vi "Offset by dx and dy.vi"(8 "error in (no error)":errorcluster caption="错误输入（无错误）", 9 "dy":dbl, 10 "dx":dbl, 11 "Point 输入":refnum<class "Point.lvclass"> caption="DNL_LabVIEW Object in") -> (0 "error out":errorcluster caption="错误输出", 3 "Point 输出":refnum<class "Point.lvclass"> caption="DNL_LabVIEW Object out")   [LabVIEW 2011, in "Point.lvclass"]
uses:
  Point.lvclass
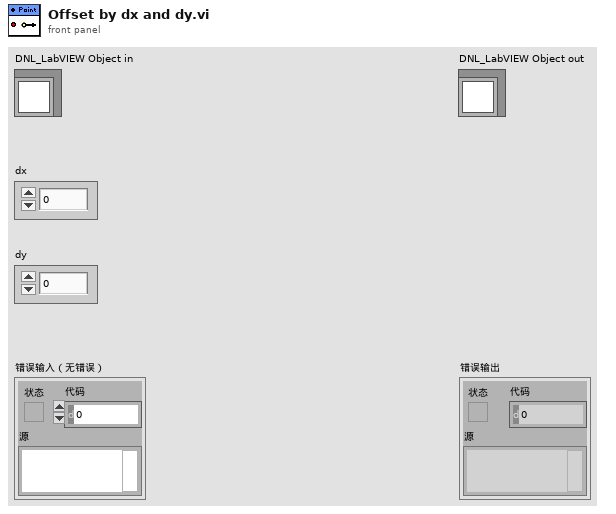
[diagram p1: front panel]
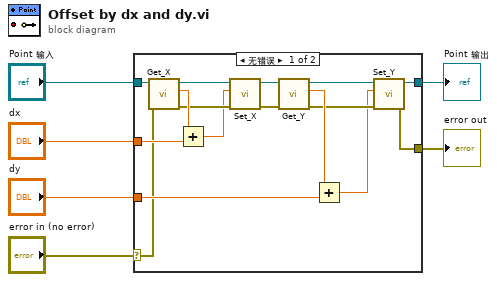
[diagram p0: block diagram]
diagram:
  n1 = case shown="无错误" "error in (no error)" {
    selector: "error in (no error)" -> [w8 w24]
    tunnel: [w7 w24] -> w5
    tunnel: [w10 w23] -> w3
    tunnel: "Point 输入" -> [w22 w23]
    tunnel: "dx" -> [w20 _]
    tunnel: "dy" -> [w15 _]
    frame No Error {
      n2 = call "Get_X.vi"("error in (no error)"=w8, "Point输入"=w22) -> ("error out"=w19:errorcluster, "X"=w21:dbl, "Point输出"=w17:refnum<class "Point.lvclass">)  [unwired: 7 in]
      n3 = Add(x=w21, y=w20) -> (x+y=w18:dbl)
      n4 = call "Set_X.vi"("error in (no error)"=w19, "X"=w18, "Point输入"=w17) -> ("error out"=w13:errorcluster, "Point输出"=w16:refnum<class "Point.lvclass">)  [unwired: 7 in]
      n5 = call "Get_Y.vi"("error in (no error)"=w13, "Point输入"=w16) -> ("error out"=w11:errorcluster, "Y"=w14:dbl, "Point输出"=w12:refnum<class "Point.lvclass">)  [unwired: 7 in]
      n6 = Add(x=w14, y=w15) -> (x+y=w9:dbl)
      n7 = call "Set_Y.vi"("error in (no error)"=w11, "Y"=w9, "Point输入"=w12) -> ("error out"=w7:errorcluster, "Point输出"=w10:refnum<class "Point.lvclass">)  [unwired: 7 in]
    }
    frame Error {
    }
  }
  "error out" <- w5
  "Point 输出" <- w3
